vi "byebye.vi"(8 "error in (no error)":errorcluster, 10 "root":T1, 11 "connection ID":refnum<k16>) -> (0 "error out":errorcluster, 3 "connection ID out":refnum<k16>)   [LabVIEW 2010]
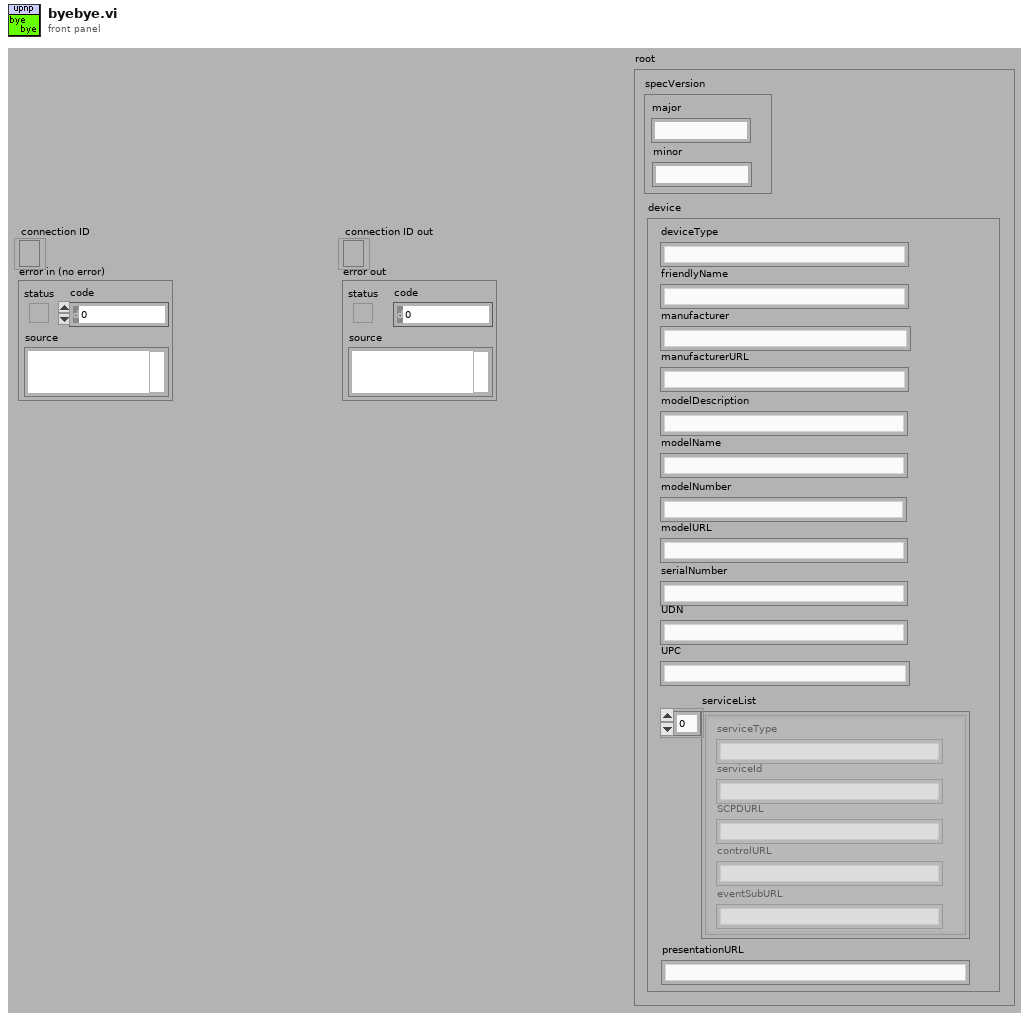
[diagram p1: front panel]
types:
  T1 = cluster{"specVersion":cluster{"major":string, "minor":string}, "device":cluster{"deviceType":string, "friendlyName":string, "manufacturer":string, "manufacturerURL":string, "modelDescription":string, "modelName":string, "modelNumber":string, "modelURL":string, "serialNumber":string, "UDN":string, "UPC":string, "serviceList":cluster{"serviceType":string, "serviceId":string, "SCPDURL":string, "controlURL":string, "eventSubURL":string}[], "presentationURL":string}}
  T2 = cluster{"serviceType":string, "serviceId":string, "SCPDURL":string, "controlURL":string, "eventSubURL":string}[]
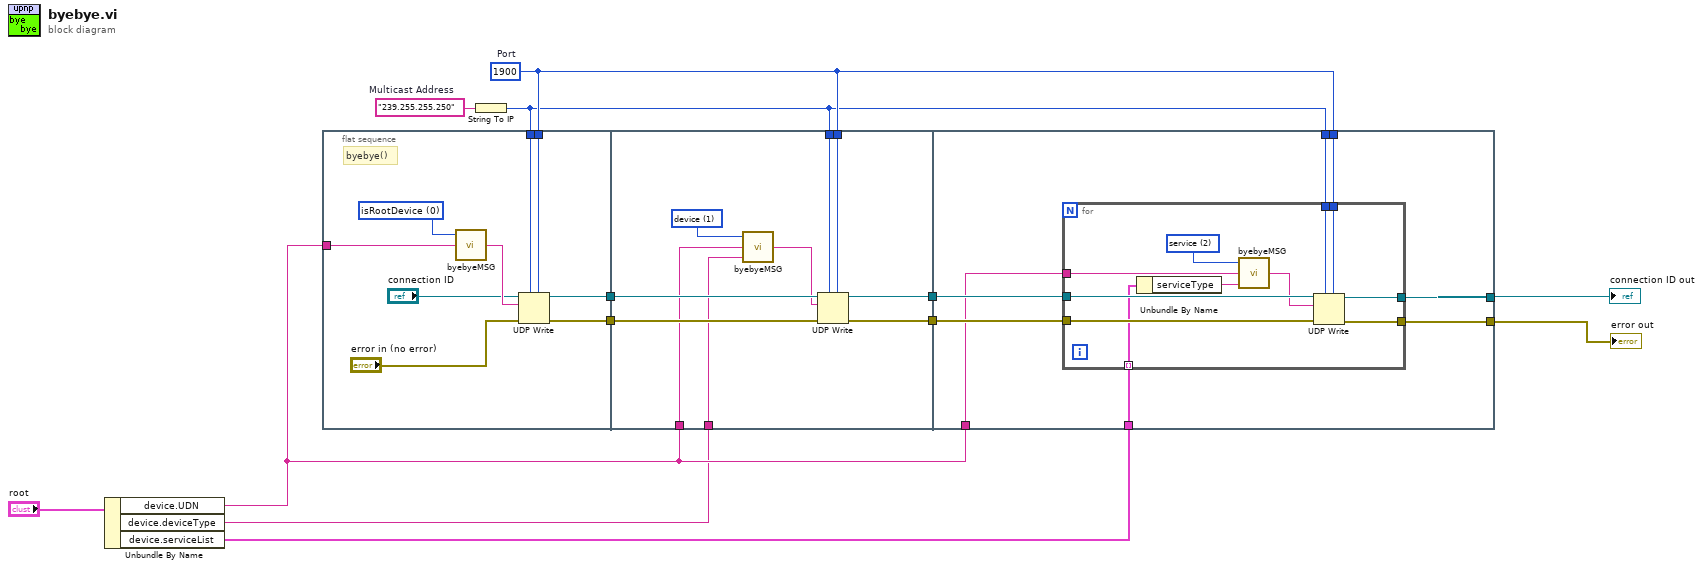
[diagram p0: block diagram]
diagram:
  w8 = u16 1900  # Port
  w9 = "239.255.255.250"  # Multicast Address
  n1 = Unbundle By Name("root") -> ("device.UDN"=w3:string, "device.deviceType"=w1:string, "device.serviceList"=w2:T2)
  n2 = flat-sequence {
    tunnel: [w21] -> w13
    tunnel: [w20] -> w12
    tunnel: w8 -> [w19]
    tunnel: w7 -> [w18]
    tunnel: w3 -> [w14]
    tunnel: w13 -> [w31]
    tunnel: w12 -> [w29]
    tunnel: [w28] -> w11
    tunnel: [w27] -> w10
    tunnel: w8 -> [w26]
    tunnel: w7 -> [w25]
    tunnel: w3 -> [w24]
    tunnel: w1 -> [w23]
    tunnel: w11 -> [w40]
    tunnel: w10 -> [w39]
    tunnel: w8 -> [w38]
    tunnel: w7 -> [w37]
    tunnel: [w36] -> w6
    tunnel: [w35] -> w5
    tunnel: w3 -> [w34]
    tunnel: w2 -> [w33]
    frame #0 {
      w15 = u16 0 items=["isRootDevice", "device", "service"] ("type of announce")
      # "byebye()"
      n3 = call "byebyeMSG.vi"("UDN"=w14, "type of announce"=w15) -> ("byebyeMSG"=w22:string)  [unwired: 1 in]
      n4 = UDP Write(address=w18, port or service name=w19, connection ID="connection ID", data in=w22, 8:"error in (no error)") -> (error out=w20:errorcluster, 3:w21:refnum<k16>)  [unwired: 1 out]
    }
    frame #1 {
      w32 = u16 1 items=["isRootDevice", "device", "service"] ("type of announce")
      n5 = call "byebyeMSG.vi"("input"=w23, "UDN"=w24, "type of announce"=w32) -> ("byebyeMSG"=w30:string)
      n6 = UDP Write(address=w25, port or service name=w26, connection ID=w31, data in=w30, 8:w29) -> (error out=w27:errorcluster, 3:w28:refnum<k16>)  [unwired: 1 out]
    }
    frame #2 {
      n7 = for {
        tunnel: w40 -> [w50]
        tunnel: w39 -> [w49]
        tunnel: w38 -> [w47]
        tunnel: w37 -> [w46]
        tunnel: [w45] -> w36
        tunnel: [w44] -> w35
        tunnel: w34 -> [w43]
        tunnel: w33 -> [w42] mode=indexing
        w51 = u16 2 items=["isRootDevice", "device", "service"] ("type of announce")
        n8 = Unbundle By Name(w42) -> ("serviceType"=w41:string)
        n9 = call "byebyeMSG.vi"("input"=w41, "UDN"=w43, "type of announce"=w51) -> ("byebyeMSG"=w48:string)
        n10 = UDP Write(address=w46, port or service name=w47, connection ID=w50, data in=w48, 8:w49) -> (error out=w44:errorcluster, 3:w45:refnum<k16>)  [unwired: 1 out]
      }
    }
  }
  n11 = String To IP(1:w9) -> (0:w7:u32)
  "connection ID out" <- w6
  "error out" <- w5
